vi "dfd_Check Subband Signals (Wfm).vi"(8 "error in (no error)":errorcluster, 11 "subband signals":waveform(dbl)[](array[waveform])) -> (0 "error out":errorcluster, 3 "dup subband signals":waveform(dbl)[](array[waveform]))   [LabVIEW 2017, in "NI_DigFilter_FilterBank.lvlib"]
uses:
  <vilib>/addons/Digital Filter Design/NI_DigFilter_FilterBank.lvlib
  <vilib>/addons/Digital Filter Design/_Misc.llb/dfd_Error Handlers (Single).vi
  <vilib>/addons/Digital Filter Design/NI_DigFilterLicensed.lvlib
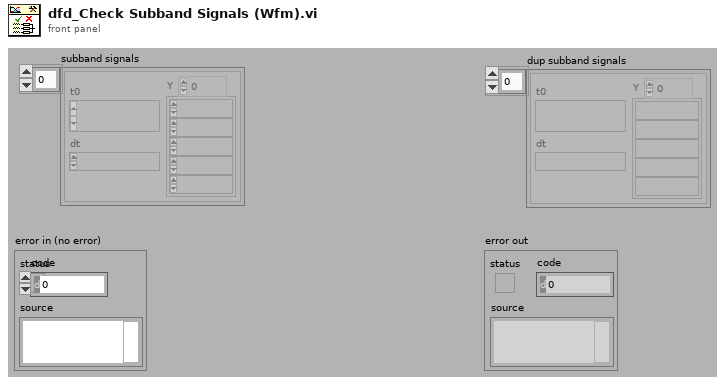
[diagram p1: front panel]
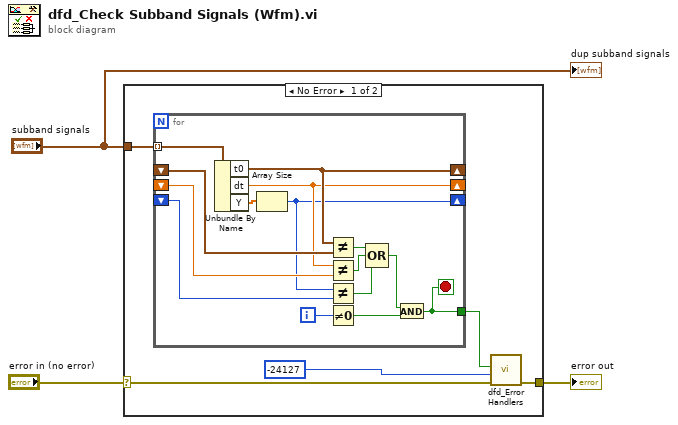
[diagram p0: block diagram]
diagram:
  n1 = case shown="No Error" "error in (no error)" {
    selector: "error in (no error)" -> [w6 w24]
    tunnel: [w7 w24] -> w2
    tunnel: "subband signals" -> [w5 _]
    frame No Error {
      n2 = for {
        tunnel: w5 -> [w22] mode=indexing
        shift-right: [w21] -> _
        shift-left: _ -> [w20]
        shift-right: [w13] -> _
        shift-left: _ -> [w19]
        tunnel: [w14] -> w4
        shift-right: [w11] -> _
        shift-left: _ -> [w10]
        i -> [w23]
        stop <- w14 stop-if-true
        n3 = Unbundle By Name(w22) -> ("t0"=w21:timestamp, "dt"=w13:dbl, "Y"=w12:dbl[])
        n4 = Array Size(array=w12) -> (size(s)=w11:i32)
        n5 = Not Equal?(x=w21, y=w20) -> (x != y?=w17:bool)
        n6 = Not Equal?(x=w13, y=w19) -> (x != y?=w16:bool)
        n7 = Not Equal?(x=w11, y=w10) -> (x != y?=w9:bool)
        n8 = Not Equal To 0?(x=w23) -> (x != 0?=w18:bool)
        n9 = Compound Arithmetic op=OR(w17, w16, w9) -> (w15:bool)
        n10 = And(x=w15, y=w18) -> (x .and. y?=w14:bool)
      }
      n11 = call-poly <vilib>:"dfd_Error Handlers.vi"("error in (no error)"=w6, "error code"=-24127 ("ERR_INVALID_SUBBAND_SIGNALS"), "condition failed?"=w4) -> ("error out"=w7:errorcluster)  [unwired: 8 in]
    }
    frame Error {
    }
  }
  "error out" <- w2
  "dup subband signals" <- "subband signals"
